vi "NichtlinearerRegler.vi"(8 "p'":dbl, 9 "p":dbl, 10 "x'":dbl) -> (2 "s? t:f":dbl)   [LabVIEW 2013]
uses:
  <vilib>/express/express arith-compare/Formula/XNode/ExpressFormulaBlockNode.xnode
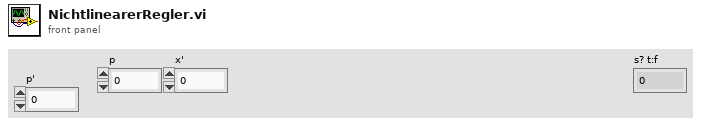
[diagram p1: front panel]
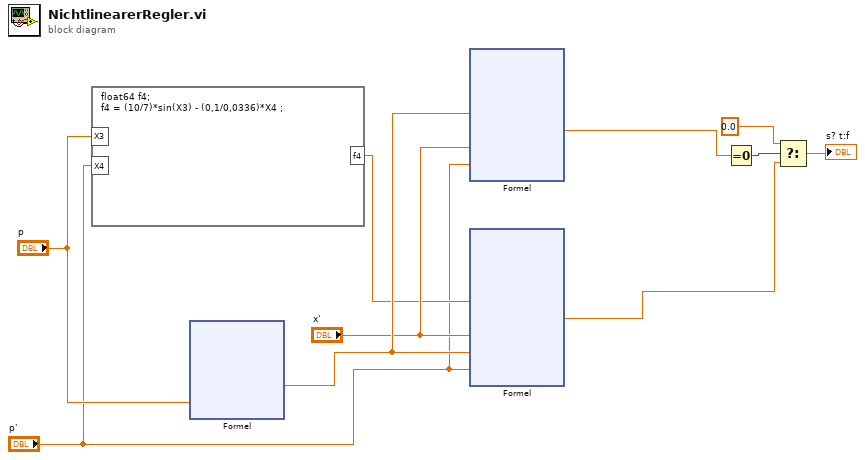
[diagram p0: block diagram]
diagram:
  n1 = formula code="float64 f4;\nf4 = (10/7)*sin(X3) - (0,1/0,0336)*X4 ;" ("Formelknoten")("X3"="p", "X4"="p'") -> ("f4"=w4:dbl)
  n2 = xnode "Formel"("X3"="p") -> ("Ergebnis"=w6:dbl)  [unwired: 1 in, 1 out]
  n3 = xnode "Formel"("g4"=w6, "X2"="x'", "X4"="p'") -> ("Ergebnis"=w7:dbl)  [unwired: 1 in, 1 out]
  n4 = xnode "Formel"("f4"=w4, "X2"="x'", "g4"=w6, "X4"="p'") -> ("Ergebnis"=w1:dbl)  [unwired: 1 in, 1 out]
  n5 = Equal To 0? ("Gleich 0?")(x=w7) -> (x = 0?=w10:bool)
  n6 = Select ("Auswählen")(t=0.0 ("value below threshold 2"), s=w10, f=w1) -> (s? t:f=→"s? t:f":dbl)
